vi "Main_v6.vi"() -> ()   [LabVIEW 2018]
uses:
  Clusters/FileDataChannel.ctl
  <vilib>/Platform/TimedLoop/XDataNode/timing_clust.ctl
  <vilib>/Platform/TimedLoop/XDataNode/nitl_modes.ctl
  <vilib>/Platform/TimedLoop/XDataNode/wakeup.ctl
  Clusters/IOSignals.ctl
  Clusters/SimulationConstants.ctl
  Clusters/RoscoParams.ctl
  Clusters/ArrayPairs.ctl
  Clusters/SwapArrayCluster.ctl
  <vilib>/Analysis/baseanly.llb/Mean (DBL).vi
  <vilib>/Utility/file.llb/Read Delimited Spreadsheet (DBL).vi
  <vilib>/Platform/TimedLoop/XDataNode/loadnilvce.vi
  <vilib>/platform/TimedLoop/XDataNode/XDataNode.xnode
  <vilib>/Platform/TimedLoop/XDataNode/XDNodeRunTimeDep.lvlib
  <vilib>/Analysis/NI_AALBase.lvlib
  <vilib>/ptbypt/NI_PtbyPt.lvlib
  <resource>/objmgr/IndComECAT.rc
  <vilib>/indcomecat/Remote IO/NI ECAT Remote IO.lvlib
panel:
  out "State logic late?":bool
  out "Actual shaft Speed (rpm)":dbl(knob)=7.068579725455493e-05 scale=-300.0..300.0
  out "Pitch setpoint (eCAT)":i32
  in  "Man Vel Set":dbl
  in  "Pitch I-Gain":dbl
  in  "Pitch P-Gain":dbl
  out "Main Gen Bus":u16 format="%.0x"
  out "Axis 3 Fault":bool
  out "Axis 3 Warning":bool
  out "Axis 2 Fault":bool
  out "Axis 2 Warning":bool
  out "Axis 1 Fault":bool
  out "Axis 1 Warning":bool
  out "Axis 3 Operational":bool
  out "Axis 2 Operational":bool
  out "Axis 1 Operational":bool
  out "Pitch Axis 3":string
  out "Pitch Axis 2":string
  out "Pitch Axis 1":string
  in  "Clear Pitch Actuator Faults (x3)":bool
  in  "Enable Pitch Actuators (x3)":bool
  out "Pitch Angle (deg) - Blade 3":dbl(knob) scale=0.0..30.0 scale format="%.2f"
  out "Pitch Angle (deg) - Blade 2":dbl(knob) scale=0.0..30.0 scale format="%.2f"
  out "Pitch Angle (deg) - Blade 1":dbl(knob) scale=0.0..30.0 scale format="%.2f"
  in  "Manual Torque":i16(slide) scale=-100.0..250.0
  out "Generator Operational":bool
  in  "Clear Accelnet Faults":bool
  in  "Enable Accelnet":bool
  out "Generator Fault":bool
  out "Generator Warning":bool
  out "Main generator state":string
  out "Rosco Failed?":bool
  in  "WS Freq (Hz)":dbl=0.009999999776482582
  in  "WS Mean":dbl=10.0
  in  "WS Amplitude":dbl
  out "Generator Torque (MNm)":dbl(knob) scale=0.0..35.0
  out "OUT_ROTSP":dbl
  out "OUT_AEROTQ":dbl
  out "SIM-Cp":dbl
  out "Generator Speed (rpm)":dbl(knob)=7.068579725455493e-05 scale=0.0..10.0
  in  "?":T1(tab)
  out "Generator Speed":dynamicdata(graph)
  out "Torque  (MNm)":dynamicdata(graph)
  out "Pitch (deg)":dynamicdata(graph)
  out "Aero Torque":dynamicdata(graph)
  out "WindSpeed(m/s)":dbl(graph)
  in  "To VS_ControlMode":T2(ring)
  in  "Edit DISCON":bool
  out "DISCON.IN Contents":string
  in  "From VS_ControlMode":T2(ring)
  out "Rosco Return Message":string
  out "Generator  Power (kW)":dbl(graph)
  out "Pitch axis 3 ctrl word":u16 format="%x"
  out "Pitch axis 2 ctrl word":u16 format="%x"
  out "avrSWAP":sgl[](array[numeric])
  out "OUT_DEBUG":dbl
  out "RT Loop Duration":i64
  out "Control Mode - Main Gen":u8
  out "WriteSDO Abort - Main Gen":u32
  out "ReadSDO Abort - Main Gen":u32
  out "Gen ctrl word":u16 format="%x"
  out "Pitch axis 1 ctrl word":u16 format="%x"
  out "Graphics Update t (s)":dbl format="%.1f"
  out "Effective rate (ms)":dbl format="%#.1f"
  out "WriteSDO Abort - Pitch 1":u32
  out "ReadSDO Abort - Pitch 1":u32
  out "Control Mode - Pitch 1":u8
  in  "Zero Pitch 1":bool
  in  "Zero Pitch 2":bool
  in  "Zero Pitch 3":bool
  out "Torque Setpoint (MNm)":dbl(knob) scale=0.0..35.0
  out "Collective pitch Setpoint (deg)":dbl(knob) scale=0.0..30.0 scale format="%.2f"
  out "Power (kW)":dbl(slide) scale=0.0..20.0 scale format="%.2f"
  out "SimLoop Late?":bool
  out "FIFO Loop Late?":bool
  in  "Base filename":string="rosco-tests"
  out "Writing to cRIO?":bool
  in  "WriteData":bool
  in  "?":T3
  out "#RT FIFO":u32
  in  "?":bool
  out "Time(s)":dbl format="%6.1g"
  out "RT Loop Late?":bool
  # "FOCAL Campaign 1"
  # "ROSCO"
  # "Processed quantities"
  # "GENERATOR INPUTS"
  # "PITCH ACTUATORS"
  # "FILEWRITING"
  # "MAIN GEN CONTROL"
  # "TEMP"
  # "PITCH ACTUATORS CONTROL"
  # "Axis 1"
  # "Axis 2"
  # "Axis 3"
  # "Operational"
  # "Warning"
  # "Error"
  # "TURBINE SPECIFICATIONS"
  # "RATED POWER: 15000000 W"
  # "RATED TORQUE: 19624046.66 Nm"
  # "RATED GEN SPEED: 0.79168 rad/s"
  # "ROSCO INPUTS"
  # "SYSTEM"
  # "ROSCO"
  # "MAIN MOTOR"
  # "PITCH AXIS 1"
  # "PITCH AXIS 2"
  # "PITCH AXIS 3"
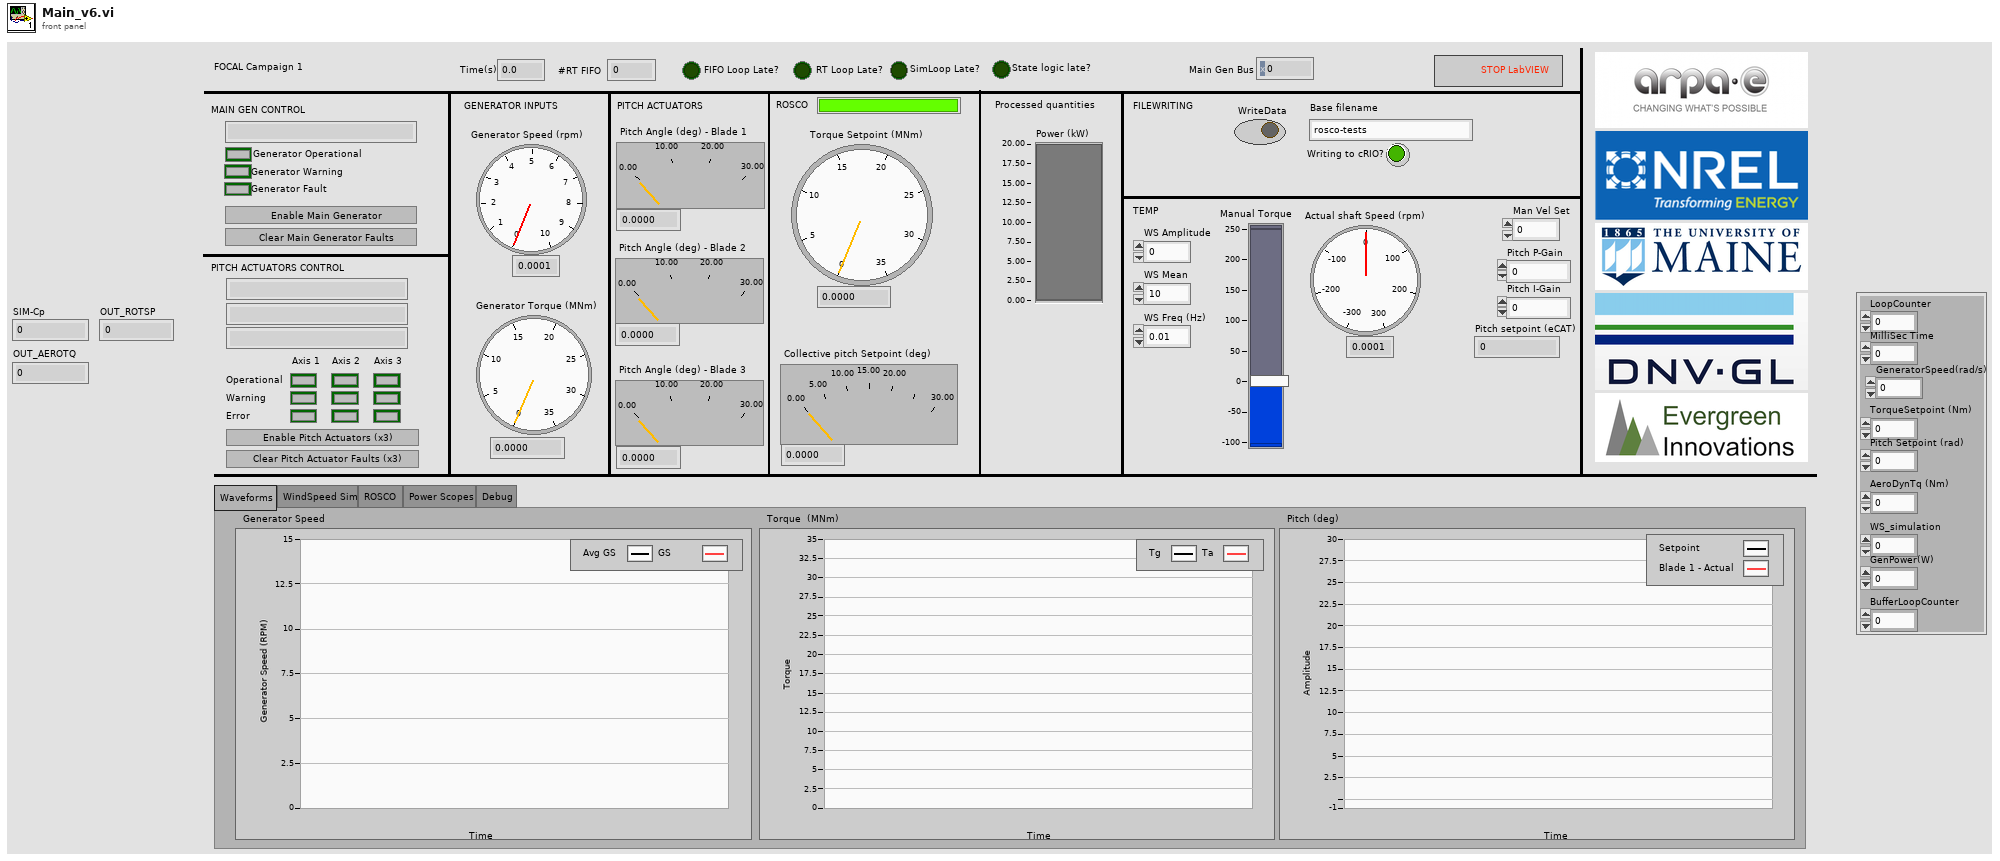
[diagram p1: front panel]
types:
  T1 = enum32{"Waveforms", "WindSpeed Sim", "ROSCO", "Power Scopes", "Debug"}
  T2 = enum16{"Constant Torque", "Constant Power", "PI Control"}
  T3 = typedef "FileDataChannel.ctl" = cluster{"GeneratorSpeed(rad/s)":dbl, "BufferLoopCounter":dbl, "LoopCounter":dbl, "TorqueSetpoint (Nm)":dbl, "Pitch Setpoint (rad)":dbl, "AeroDynTq (Nm) ":dbl, "WS_simulation":dbl, "GenPower(W)":dbl, "MilliSec Time ":dbl}
  T4 = typedef "IOSignals.ctl" = cluster{"mainGenPosition (rev)":dbl, "mainGenTorque (Nm)":dbl, "mainGenVelocity (rpm)":dbl, "mainGenStatus":u16, "pitch1Position (rev)":dbl, "pitch1Velocity (rev/s)":dbl, "pitch1Status":u16, "pitch2Position (rev)":dbl, "pitch2Velocity (rev/s)":dbl, "pitch2Status":u16, "pitch3Position (rev)":dbl, "pitch3Velocity (rev/s)":dbl, "pitch3Status":u16, "pitch1PosOfst (rev)":dbl, "pitch2PosOfst (rev)":dbl, "pitch3PosOfst (rev)":dbl}
  T5 = typedef "ArrayPairs.ctl" = cluster{"iStatus":T6, "TIME":T6, "DT":T6, "BL_PITCH":T6, "VS_MECHGENPWR":T6, "VS_GENPWR":T6, "GEN_SPEED":T6, "ROTOR_SPEED":T6, "GENTQMEAS":T6, "Y_M":T6, "HORWINDV":T6, "ROOTMOOP1":T6, "ROOTMOOP2":T6, "BL_PITCH2":T6, "BL_PITCH3":T6, "ROOTMOOP3":T6, "AVCMSG_SIZE":T6, "INFILE_SIZE ":T6, "OUTFILE_SIZE ":T6, "FA_ACC":T6, "NUM_BLADES":T6, "OUT_BL_PITCH":T6, "OUT_TORQUE":T6, "OUT_AEROTQ":T6, "Out.RotSpeed ":T6, "Out.DEBUG":T6}
  T6 = typedef "SwapArrayCluster.ctl" = cluster{"Index":i32, "Value":dbl}
  T7 = typedef "RoscoParams.ctl" = cluster{"avrSWAP":sgl[], "aviFAIL":i32, "avcMSG":string, "ReturnValue":i32}
  T8 = typedef "XDNodeRunTimeDep.lvlib/timing_clust.ctl" = cluster{"Expected End [f-1]":u64, "Actual End [f-1]":u64, "Finished Late? [f-1]":bool, "Expected End [i-1]":u64, "Actual End [i-1]":u64, "Finished Late? [i-1]":bool, "Expected Start [i]":u64, "Actual Start [i]":u64, "Expected Start [f]":u64, "Actual Start [f]":u64, "Source Name":string, "Structure Name":string, "Period":i64, "Deadline":i64, "Offset":i64, "Start":i64, "Priority":i32, "Timeout":i32, "Mode":T9, "Wakeup Reason":T10, "Error":errorcluster, "Source Type":string, "Secondary Source Type":string, "Global End Time":u64, "Global Start Time":u64, "Frame Duration":u64, "Iteration Duration":u64, "Assigned CPU":i32, "I/O Scan Engine Mode":u32}
  T9 = typedef "XDNodeRunTimeDep.lvlib/nitl_modes.ctl" = enum32{"No Change", "Process missed periods, maintain original phase", "Discard missed periods, maintain original phase", "Process missed periods, ignore original phase", "Discard missed periods, ignore original phase"}
  T10 = typedef "XDNodeRunTimeDep.lvlib/wakeup.ctl" = enum32{"Normal", "Aborted", "Asynchronous wakeup", "Timing source error", "Timed loop error", "Timeout"}
  T11 = typedef "SimulationConstants.ctl" = cluster{"Ngear":dbl, "RotorInertia":dbl, "GeneratorEff":dbl, "RotorRadius":sgl, "Rho":dbl, "NumBlades":dbl, "AVCMSG_SIZE":dbl}
  T12 = typedef "ElmoState.ctl" = cluster{"Elmo State":string, "Elmo Operational":bool, "Elmo Warning":bool, "Elmo Fault":bool}
  T13 = typedef "AccelnetState.ctl" = cluster{"State String":string, "Accelnet Warning":bool, "Accelnet Fault":bool, "Accelnet Operational":bool}
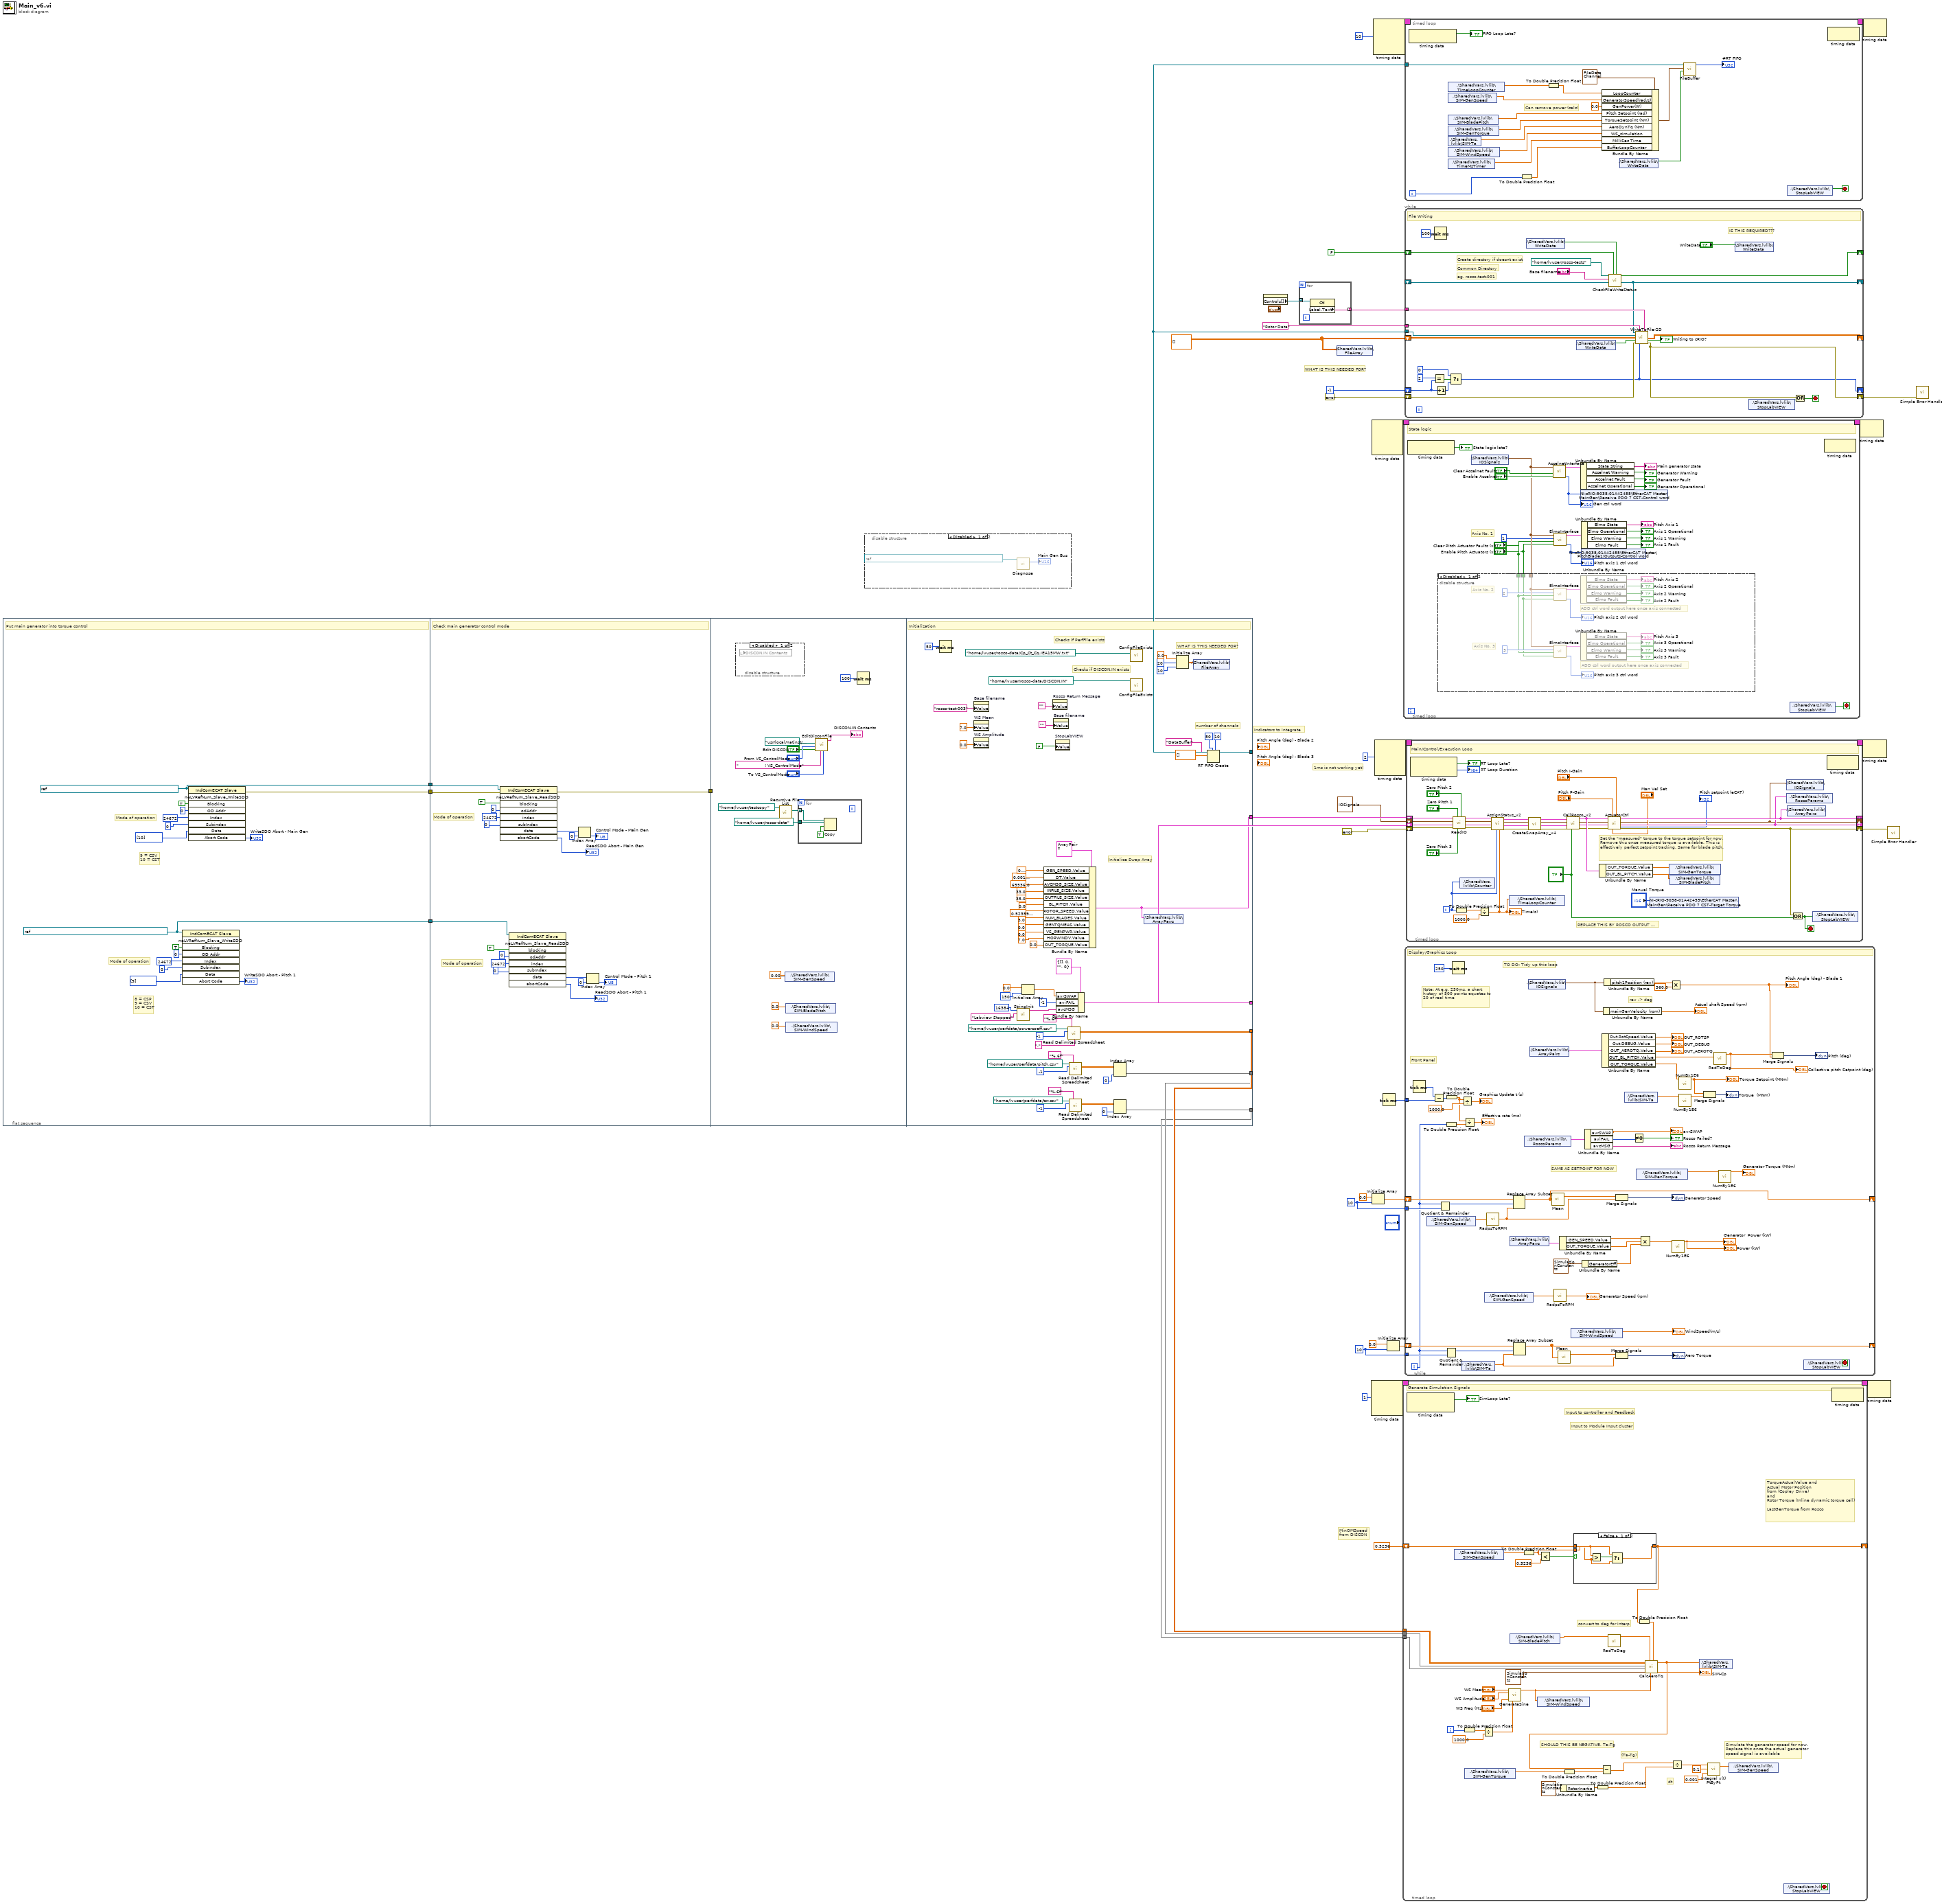
[diagram p0: block diagram]
diagram:
  w16 = 10 ("dimension size")
  w13 = 10 ("dimension size")
  w31 = dbl[][] [] ("File array 2")
  # "Indicators to integrate"
  # "WHAT IS THIS NEEDED FOR?"
  # "1ms is not working yet!"
  # "MinOMSpeed\nfrom DISCON"
  n1 = flat-sequence {
    tunnel: [w48] -> w10
    tunnel: [w49] -> w9
    tunnel: [w41] -> w1
    tunnel: w10 -> [w67]
    tunnel: w9 -> [w66]
    tunnel: [w65] -> w8
    tunnel: w1 -> [w56]
    tunnel: w8 -> [_]
    tunnel: [w140] -> w4
    tunnel: [w129] -> w24
    tunnel: [w105] -> w23
    tunnel: [w118] -> w22
    tunnel: [w117] -> w21
    tunnel: [w92] -> w15
    frame #0 {
      w41 = refnum<k21> "ni.var.io://ni-crio-9038-01a42455/EtherCAT Master/PitchBlade1" ("Slave Constant")
      w48 = refnum<k21> "ni.var.io://ni-crio-9038-01a42455/EtherCAT Master/MainGen" ("Slave Constant")
      # "Mode of operation"
      # "8 = CSP \n9 = CSV\n10 = CST"
      # "Mode of operation"
      # "9 = CSV\n10 = CST"
      # "Put main generator into torque control"
      n2 = invoke class="IndComECAT Slave" method="neLVRefNum_Slave_WriteSDO"(reference=w41, "Blocking"=TRUE, "OD Addr"=u16 0, "Index"=u16 24672, "Subindex"=u8 0, "Data"=u8[] [9]) -> ("Abort Code"=→"WriteSDO Abort - Pitch 1":u32)  [unwired: 3 in, 8 out]
      n3 = invoke class="IndComECAT Slave" method="neLVRefNum_Slave_WriteSDO"(reference=w48, "Blocking"=TRUE, "OD Addr"=u16 0, "Index"=u16 24672, "Subindex"=u8 0, "Data"=u8[] [10]) -> (error out=w49:errorcluster, "Abort Code"=→"WriteSDO Abort - Main Gen":u32)  [unwired: 3 in, 7 out]
    }
    frame #1 {
      # "Mode of operation"
      # "Mode of operation"
      # "Check main generator control mode"
      n4 = invoke class="IndComECAT Slave" method="neLVRefNum_Slave_ReadSDO"(reference=w67, error in=w66, "blocking"=TRUE, "odAddr"=u16 0 ("OD address"), "index"=u16 24672 ("Index"), "subIndex"=u8 0 ("Subindex")) -> (error out=w65:errorcluster, "data"=w70:u8[], "abortCode"=→"ReadSDO Abort - Main Gen":u32)  [unwired: 3 in, 6 out]
      n5 = invoke class="IndComECAT Slave" method="neLVRefNum_Slave_ReadSDO"(reference=w56, "blocking"=TRUE, "odAddr"=u16 0 ("OD address"), "index"=u16 24672 ("Index"), "subIndex"=u8 0 ("Subindex")) -> ("data"=w59:u8[], "abortCode"=→"ReadSDO Abort - Pitch 1":u32)  [unwired: 4 in, 7 out]
      n6 = Index Array(array=w70, index=0) -> (element=→"Control Mode - Main Gen":u8)
      n7 = Index Array(array=w59, index=0) -> (element=→"Control Mode - Pitch 1":u8)
    }
    frame #2 {
      n8 = disable-structure shown="Disabled" {
        frame Disabled {
          n9 = local read "DISCON.IN Contents"() -> ()  [unwired: 1 in]
        }
        frame Enabled {
        }
      }
      n10 = call <vilib>:"Recursive File List.vi"("Folder Path"=path "/home/lvuser/testcopy" ("path")) -> ("All Files in Dir"=w78:path[])  [unwired: 6 in, 4 out]
      n11 = shared-variable ".\\SharedVars.lvlib\\SIM-GenSpeed"(0.009999999776482582 ("RotorSpeed(rad/s)")) -> ()  [unwired: 1 in, 1 out]
      n12 = shared-variable ".\\SharedVars.lvlib\\SIM-BladePitch"(0.0 ("ecat-BladePitch")) -> ()  [unwired: 1 in, 1 out]
      n13 = shared-variable ".\\SharedVars.lvlib\\SIM-WindSpeed"(0.0 ("WindSpeedSim")) -> ()  [unwired: 1 in, 1 out]
      n14 = for {
        tunnel: path "/home/lvuser/rosco-data" ("target path (use dialog)") -> [w91]
        tunnel: w78 -> [w90] mode=indexing
        n15 = Copy(9:TRUE ("overwrite (F)"), 10:w91, 11:w90) -> ()  [unwired: 2 in, 3 out]
      }
      n16 = call "EditDisconFile.vi"("To VS_ControlMode"="To VS_ControlMode", "Append"="                   ! VS_ControlMode", "Edit DISCON"="Edit DISCON", "From VS_ControlMode"="From VS_ControlMode", "path"=path "/usr/local/natinst/labview/DISCON.IN") -> ("data"=→"DISCON.IN Contents":string)  [unwired: 4 in, 1 out]
      n17 = Wait (ms)(milliseconds to wait=u32 100) -> ()  [unwired: 1 out]
    }
    frame #3 {
      # "WHAT IS THIS NEEDED FOR?"
      # "number of channels"
      # "Checks if PerfFile exists"
      # "Checks if DISCON.IN exists"
      # "Initialize Swap Array"
      # "Initialization"
      n18 = Wait (ms)(milliseconds to wait=u32 50) -> ()  [unwired: 1 out]
      n19 = property on="Base filename" class="Str"("Value"="rosco-test-003" ("Base filename")) -> ()  [unwired: 2 in, 2 out]
      n20 = property on="WS Mean" class="DigNum (strict)"("Value"=7.0 ("GenSpeed Mean")) -> ()  [unwired: 2 in, 2 out]
      n21 = property on="WS Amplitude" class="DigNum (strict)"("Value"=0.0 ("GenSpeeed Amplitude")) -> ()  [unwired: 2 in, 2 out]
      n22 = call "StringInit.vi"("accOUTNAME"="Labview Stopped", "dimension size"=16384) -> ("result string"=w144:string)  [unwired: 9 in]
      n23 = Initialize Array(sgl 0.0 ("element"), 150 ("dimension size")) -> (w98:sgl[])
      n24 = Bundle By Name(cluster=T5 {"iStatus"={"Index"=0, "Value"=0.0}, "TIME"={"Index"=1, "Value"=0.0}, "DT"={"Index"=2, "Value"=0.0}, "BL_PITCH"={"Index"=3, "Value"=0.0}, "VS_MECHGENPWR"={"Index"=13, "Value"=0.0}, "VS_GENPWR"={"Index"=14, "Value"=0.0}, "GEN_SPEED"={"Index"=19, "Value"=0.0}, "ROTOR_SPEED"={"Index"=20, "Value"=0.0}, "GENTQMEAS"={"Index"=22, "Value"=0.0}, "Y_M"={"Index"=23, "Value"=0.0}, "HORWINDV"={"Index"=26, "Value"=0.0}, "ROOTMOOP1"={"Index"=29, "Value"=0.0}, "ROOTMOOP2"={"Index"=30, "Value"=0.0}, "BL_PITCH2"={"Index"=32, "Value"=0.0}, "BL_PITCH3"={"Index"=33, "Value"=0.0}, "ROOTMOOP3"={"Index"=31, "Value"=0.0}, "AVCMSG_SIZE"={"Index"=48, "Value"=0.0}, "INFILE_SIZE "={"Index"=49, "Value"=0.0}, "OUTFILE_SIZE "={"Index"=50, "Value"=0.0}, "FA_ACC"={"Index"=52, "Value"=0.0}, "NUM_BLADES"={"Index"=60, "Value"=0.0}, "OUT_BL_PITCH"={"Index"=44, "Value"=0.0}, "OUT_TORQUE"={"Index"=46, "Value"=0.0}, "OUT_AEROTQ"={"Index"=91, "Value"=0.0}, "Out.RotSpeed "={"Index"=92, "Value"=0.0}, "Out.DEBUG"={"Index"=93, "Value"=0.0}} ("ArrayPairs"), "GEN_SPEED.Value"=0.30000001192092896 ("GeneratorSpeed(rad/s)"), "DT.Value"=0.0010000000474974513 ("Dt"), "AVCMSG_SIZE.Value"=65536.0 ("new element/subarray"), "INFILE_SIZE.Value"=33.0 ("new element/subarray"), "OUTFILE_SIZE.Value"=35.0 ("new element/subarray"), "BL_PITCH.Value"=0.0 ("GeneratorTorque(Nm)"), "ROTOR_SPEED.Value"=0.5235999822616577 ("RotorSpeed(rad/s)"), "NUM_BLADES.Value"=3.0 ("NumberofBlades"), "GENTQMEAS.Value"=0.0 ("BladePitch(rad)"), "VS_GENPWR.Value"=0.0 ("Generator Power(W)"), "HORWINDV.Value"=7.0 ("WindSpeed(m/s)"), "OUT_TORQUE.Value"=0.0) -> (w92:T5)
      n25 = property on="Rosco Return Message" class="Str"("Value"="") -> ()  [unwired: 2 in, 2 out]
      n26 = property on="Base filename" class="Str"("Value"="") -> ()  [unwired: 2 in, 2 out]
      n27 = property on="StopLabVIEW" class="Bool (strict)"("Value"=FALSE) -> ()  [unwired: 2 in, 2 out]
      n28 = Bundle By Name(cluster=T7 {"avrSWAP"=[], "aviFAIL"=0, "avcMSG"="", "ReturnValue"=0}, "avrSWAP"=w98, "aviFAIL"=-1, "avcMSG"=w144) -> (w129:T7)
      n29 = call-poly <vilib>:"Read Delimited Spreadsheet.vi"("file path (dialog if empty)"=path "/home/lvuser/perfdata/powercoeff.csv", "format (%.3f)"="%.6f", "number of rows (all:-1)"=-1, "delimiter (\\t)"="," ("delimiter (\\t)")) -> ("all rows"=w105:dbl[][])  [unwired: 6 in, 5 out]
      n30 = call-poly <vilib>:"Read Delimited Spreadsheet.vi"("file path (dialog if empty)"=path "/home/lvuser/perfdata/pitch.csv", "format (%.3f)"="%.6f", "number of rows (all:-1)"=-1) -> ("all rows"=w122:dbl[][])  [unwired: 7 in, 5 out]
      n31 = call-poly <vilib>:"Read Delimited Spreadsheet.vi"("file path (dialog if empty)"=path "/home/lvuser/perfdata/tsr.csv", "format (%.3f)"="%.6f", "number of rows (all:-1)"=-1) -> ("all rows"=w124:dbl[][])  [unwired: 7 in, 5 out]
      n32 = Index Array(array=w122, index (col)=0 ("disabled index (col)")) -> (element=w118:dbl[])  [unwired: 1 in]
      n33 = Index Array(array=w124, index (col)=0 ("disabled index (col)")) -> (element=w117:dbl[])  [unwired: 1 in]
      n34 = call "ConfigFileExists.vi"("path"=path "/home/lvuser/rosco-data/Cp_Ct_Cq.IEA15MW.txt") -> ()  [unwired: 11 in]
      n35 = call "ConfigFileExists.vi"("path"=path "/home/lvuser/rosco-data/DISCON.IN") -> ()  [unwired: 11 in]
      n36 = shared-variable ".\\SharedVars.lvlib\\ArrayPairs"(w92) -> ()  [unwired: 1 in, 1 out]
      n37 = Initialize Array(0.0 ("element"), 20 ("dimension size"), 10 ("dimension size")) -> (w136:dbl[][])
      n38 = shared-variable ".\\SharedVars.lvlib\\FileArray"(w136) -> ()  [unwired: 1 in, 1 out]
      n39 = RT FIFO Create(0:"DataBuffer" ("name (unnamed)"), 1:dbl[] [] ("appended array"), 4:u32 50, 6:u32 10) -> (8:w140:refnum<k33>)  [unwired: 4 in, 2 out]
    }
  }
  n40 = disable-structure shown="Disabled" {
    frame Disabled {
      n41 = call <vilib>:"Diagnose.vi"("slave reference in"=refnum<k21> "ni.var.io://ni-crio-9038-01a42455/EtherCAT Master/MainGen" ("Slave Constant")) -> ("bus state"=→"Main Gen Bus":u16)  [unwired: 10 in, 4 out]
    }
    frame Enabled {
    }
  }
  n42 = property class="Clust (strict)"() -> ("Controls[]"=w34:refnum<vi>[])  [unwired: 2 in, 2 out]
  n43 = for {
    tunnel: w34 -> [w153] mode=indexing
    tunnel: [w152] -> w33 mode=indexing
    n44 = property class="Ctl"(reference=w153) -> ("Label.Text"=w152:string)  [unwired: 1 in, 2 out]
  }
  n45 = shared-variable ".\\SharedVars.lvlib\\FileArray"(w31) -> ()  [unwired: 1 in, 1 out]
  n46 = node-c288(i64 1 ("Period")) -> (w40:T8)  [unwired: 3 in]
  n47 = node-c288() -> (w12:T8)  [unwired: 4 in]
  n48 = Initialize Array(0.0 ("element"), w13) -> (w19:dbl[])
  n49 = node-c288(i64 10 ("Period")) -> (w7:T8)  [unwired: 3 in]
  n50 = node-c288(i64 2 ("Period")) -> (w38:T8)  [unwired: 3 in]
  n51 = Tick Count (ms)() -> (millisecond timer value=w2:u32)
  n52 = Initialize Array(0.0 ("element"), w16) -> (w17:dbl[])
  n53 = timed-loop {
    timing: w40 -> [_]
    timing-out: [_] -> w39
    tunnel: w23 -> [w186]
    tunnel: w22 -> [w185]
    tunnel: w21 -> [w184]
    shift-right: [w156] -> _
    shift-left: 0.5236 -> [w158]
    i -> [w167]
    stop <- w188 stop-if-true
    # "Simulate the generator speed for now. Replace this once the actual generator speed signal is available"
    # "dt"
    # "SHOULD THIS BE NEGATIVE, Ta-Tg"
    # "(Ta-Tg)"
    # "convert to deg for interp"
    # "TorqueActualValue and \nActual Motor Position \nfrom (Copley Drive)\nand\nRotor Torque (Inline dynamic torque cell)\n\nLastGenTorque from Rosco"
    # "Input to Module Input cluster"
    # "Input to controller and Feedback"
    # "Generate Simulation Signals"
    n54 = node-c288() -> (→"SimLoop Late?":bool)  [unwired: 1 in, 1 out]
    n55 = shared-variable ".\\SharedVars.lvlib\\SIM-GenSpeed"() -> (w161:dbl)  [unwired: 1 in, 1 out]
    n56 = To Double Precision Float(number=w167) -> (double precision float=w166:dbl)
    n57 = shared-variable ".\\SharedVars.lvlib\\SIM-GenTorque"() -> (w172:dbl)  [unwired: 1 in, 1 out]
    n58 = Divide(x=w166, y=1000.0) -> (x/y=w177:dbl)
    n59 = call "GenerateSine.vi"("GenSpeed Mean"="WS Mean", "GenSpeeed Amplitude"="WS Amplitude", "frequency (f)"="WS Freq (Hz)", "time (s)"=w177) -> ("sine out"=w165:dbl)  [unwired: 11 in]
    n60 = shared-variable ".\\SharedVars.lvlib\\SIM-BladePitch"() -> (w154:dbl)  [unwired: 1 in, 1 out]
    n61 = To Double Precision Float(number=w161) -> (double precision float=w157:dbl)
    n62 = shared-variable ".\\SharedVars.lvlib\\SIM-WindSpeed"(w165) -> ()  [unwired: 1 in, 1 out]
    n63 = Less?(x=w157, y=0.5236) -> (x < y?=w159:bool)
    n64 = Unbundle By Name(T11 {"Ngear"=1.0, "RotorInertia"=318628128.0, "GeneratorEff"=0.9700000286102295, "RotorRadius"=120.0, "Rho"=1.225000023841858, "NumBlades"=1.225000023841858, "AVCMSG_SIZE"=1.225000023841858} ("SimulationConst")) -> ("RotorInertia"=w175:dbl)
    n65 = To Double Precision Float(number=w172) -> (double precision float=w173:dbl)
    n66 = case shown="False" w159 {
      tunnel: [w189 w193] -> w156
      tunnel: w158 -> [w190 w193]
      tunnel: w157 -> [w191 _]
      frame False {
        n67 = Greater?(x=w191, y=w190) -> (0:w192:bool)
        n68 = Select(t=w191, s=w192, f=w190) -> (s? t:f=w189:dbl)
      }
      frame True {
      }
    }
    n69 = To Double Precision Float(number=w175) -> (double precision float=w171:dbl)
    n70 = call "RadToDeg.vi"("Double"=w154) -> ("Numeric"=w164:dbl)  [unwired: 10 in]
    n71 = To Double Precision Float(number=w156) -> (double precision float=w176:dbl)
    n72 = call "CalcAeroTq.vi"("GenSpeed"=w176, "WindSpeed"=w165, "Xi"=w164, "SimulationConst"=T11 {"Ngear"=1.0, "RotorInertia"=318628128.0, "GeneratorEff"=0.9700000286102295, "RotorRadius"=120.0, "Rho"=1.225000023841858, "NumBlades"=1.225000023841858, "AVCMSG_SIZE"=1.225000023841858}, "tsr(Y)"=w184, "pitch (X)"=w185, "Cp(Z)"=w186) -> ("Cp"=→"SIM-Cp":dbl, "Ta"=w163:dbl)  [unwired: 2 in]
    n73 = Subtract(x=w163, y=w173) -> (x-y=w162:dbl)
    n74 = Divide(x=w162, y=w171) -> (x/y=w170:dbl)
    n75 = shared-variable ".\\SharedVars.lvlib\\SIM-Ta"(w163) -> ()  [unwired: 1 in, 1 out]
    n76 = call <vilib>:"Integral x(t) PtByPt.vi"("dt"=0.001, "initial condition"=0.1, "x"=w170) -> ("integral x(t)"=w155:dbl)  [unwired: 1 in, 1 out]
    n77 = shared-variable ".\\SharedVars.lvlib\\SIM-GenSpeed"(w155) -> ()  [unwired: 1 in, 1 out]
    n78 = shared-variable ".\\SharedVars.lvlib\\StopLabVIEW"() -> (w188:bool)  [unwired: 1 in, 1 out]
    n79 = node-c288() -> ()  [unwired: 1 in, 1 out]
  }
  n80 = timed-loop {
    timing: w12 -> [_]
    timing-out: [_] -> w11
    stop <- w216 stop-if-true
    # "Axis No. 1"
    # "State logic"
    n81 = node-c288() -> (→"State logic late?":bool)  [unwired: 1 in]
    n82 = shared-variable ".\\SharedVars.lvlib\\IOSignals"() -> (w207:T4)  [unwired: 1 in, 1 out]
    n83 = disable-structure shown="Disabled" {
      disable-tunnel: w207 -> [w233 _]
      disable-tunnel: "Clear Pitch Actuator Faults (x3)" -> [w229 _]
      disable-tunnel: "Enable Pitch Actuators (x3)" -> [w228 _]
      frame Disabled {
        # "ADD ctrl word output here once axis connected"
        # "ADD ctrl word output here once axis connected"
        # "Axis No. 3"
        # "Axis No. 2"
        n84 = call "ElmoInterface.vi"("Enable"=w228, "Clear faults"=w229, "Axis No."=u32 2, "IO Signals"=w233) -> ("Control word"=→"Pitch axis 2 ctrl word":u16, "Elmo State Cluster Out"=w231:T12)  [unwired: 6 in]
        n85 = call "ElmoInterface.vi"("Enable"=w228, "Clear faults"=w229, "Axis No."=u32 3, "IO Signals"=w233) -> ("Control word"=→"Pitch axis 3 ctrl word":u16, "Elmo State Cluster Out"=w227:T12)  [unwired: 6 in]
        n86 = Unbundle By Name(w231) -> ("Elmo State"=→"Pitch Axis 2":string, "Elmo Operational"=→"Axis 2 Operational":bool, "Elmo Warning"=→"Axis 2 Warning":bool, "Elmo Fault"=→"Axis 2 Fault":bool)
        n87 = Unbundle By Name(w227) -> ("Elmo State"=→"Pitch Axis 3":string, "Elmo Operational"=→"Axis 3 Operational":bool, "Elmo Warning"=→"Axis 3 Warning":bool, "Elmo Fault"=→"Axis 3 Fault":bool)
      }
      frame Enabled {
      }
    }
    n88 = call "AccelnetInterface.vi"("Enable"="Enable Accelnet", "Clear Faults"="Clear Accelnet Faults", "IO Signals"=w207) -> ("Control word"=w211:u16, "Accelnet State"=w215:T13)  [unwired: 7 in]
    "Gen ctrl word" <- w211
    n89 = call "ElmoInterface.vi"("Enable"="Enable Pitch Actuators (x3)", "Clear faults"="Clear Pitch Actuator Faults (x3)", "Axis No."=u32 1, "IO Signals"=w207) -> ("Control word"=w198:u16, "Elmo State Cluster Out"=w206:T12)  [unwired: 6 in]
    "Pitch axis 1 ctrl word" <- w198
    n90 = Unbundle By Name(w215) -> ("State String"=→"Main generator state":string, "Accelnet Warning"=→"Generator Warning":bool, "Accelnet Fault"=→"Generator Fault":bool, "Accelnet Operational"=→"Generator Operational":bool)
    n91 = shared-variable "NI-cRIO-9038-01A42455\\EtherCAT Master\\MainGen\\Receive PDO 7 CST-Control word"(w211) -> ()  [unwired: 1 in, 1 out]
    n92 = Unbundle By Name(w206) -> ("Elmo State"=→"Pitch Axis 1":string, "Elmo Operational"=→"Axis 1 Operational":bool, "Elmo Warning"=→"Axis 1 Warning":bool, "Elmo Fault"=→"Axis 1 Fault":bool)
    n93 = shared-variable "NI-cRIO-9038-01A42455\\EtherCAT Master\\PitchBlade1\\Outputs-Control word"(w198) -> ()  [unwired: 1 in, 1 out]
    n94 = shared-variable ".\\SharedVars.lvlib\\StopLabVIEW"() -> (w216:bool)  [unwired: 1 in, 1 out]
    n95 = node-c288() -> ()  [unwired: 1 in, 1 out]
  }
  n96 = timed-loop {
    timing: w7 -> [_]
    timing-out: [_] -> w6
    tunnel: w4 -> [w238]
    i -> [w237]
    stop <- w239 stop-if-true
    # "Can remove power (calc)"
    n97 = node-c288() -> (→"FIFO Loop Late?":bool)  [unwired: 1 in]
    n98 = shared-variable ".\\SharedVars.lvlib\\TimeLoopCounter"() -> (w245:dbl)  [unwired: 1 in, 1 out]
    n99 = shared-variable ".\\SharedVars.lvlib\\SIM-GenSpeed"() -> (w253:dbl)  [unwired: 1 in, 1 out]
    n100 = shared-variable ".\\SharedVars.lvlib\\SIM-BladePitch"() -> (w247:dbl)  [unwired: 1 in, 1 out]
    n101 = shared-variable ".\\SharedVars.lvlib\\SIM-GenTorque"() -> (w248:dbl)  [unwired: 1 in, 1 out]
    n102 = shared-variable ".\\SharedVars.lvlib\\SIM-Ta"() -> (w249:dbl)  [unwired: 1 in, 1 out]
    n103 = shared-variable ".\\SharedVars.lvlib\\SIM-WindSpeed"() -> (w250:dbl)  [unwired: 1 in, 1 out]
    n104 = shared-variable ".\\SharedVars.lvlib\\TimeMsTimer"() -> (w251:dbl)  [unwired: 1 in, 1 out]
    n105 = To Double Precision Float(number=w237) -> (double precision float=w246:dbl)
    n106 = To Double Precision Float(number=w245) -> (double precision float=w240:dbl)
    n107 = Bundle By Name(cluster=T3 {"GeneratorSpeed(rad/s)"=0.0, "BufferLoopCounter"=0.0, "LoopCounter"=0.0, "TorqueSetpoint (Nm)"=0.0, "Pitch Setpoint (rad)"=0.0, "AeroDynTq (Nm) "=0.0, "WS_simulation"=0.0, "GenPower(W)"=0.0, "MilliSec Time "=0.0} ("SwapIn"), "LoopCounter"=w240, "GeneratorSpeed(rad/s)"=w253, "GenPower(W)"=0.0, "Pitch Setpoint (rad)"=w247, "TorqueSetpoint (Nm)"=w248, "AeroDynTq (Nm)"=w249, "WS_simulation"=w250, "MilliSec Time"=w251, "BufferLoopCounter"=w246) -> (w242:T3)
    n108 = shared-variable ".\\SharedVars.lvlib\\WriteData"() -> (w243:bool)  [unwired: 1 in, 1 out]
    n109 = call "FileBuffer.vi"("Boolean"=w243, "FileDataChannel"=w242, "Refnum in"=w238) -> ("# elements"=→"#RT FIFO":u32)  [unwired: 8 in]
    n110 = shared-variable ".\\SharedVars.lvlib\\StopLabVIEW"() -> (w239:bool)  [unwired: 1 in, 1 out]
    n111 = node-c288() -> ()  [unwired: 1 in, 1 out]
  }
  n112 = while {
    shift-right: [w260] -> _
    shift-left: _ -> [w261]
    shift-right: [w268] -> _
    shift-left: FALSE -> [w269]
    shift-right: [w280] -> w27
    shift-left: errorcluster {"status"=FALSE, "code"=0, "source"=""} ("error out") -> [w279]
    tunnel: "Rotor Data" -> [w263]
    tunnel: w33 -> [w264]
    tunnel: w4 -> [w265]
    shift-right: [w276] -> _
    shift-left: -1 -> [w278]
    shift-right: [w271] -> _
    shift-left: w31 -> [w277]
    stop <- w282 stop-if-true
    # "IS THIS REQUIRED???"
    # "eg. rosco-test-001"
    # "Create directory if doesnt exist"
    # "Common Directory"
    # "File Writing"
    n113 = Equal?(x=2 ("t"), y=w278) -> (x = y?=w273:bool)
    n114 = Wait (ms)(milliseconds to wait=u32 100) -> ()  [unwired: 1 out]
    n115 = Increment(x=w278) -> (x+1=w272:i32)
    n116 = Select(t=0, s=w273, f=w272) -> (s? t:f=w276:i32)
    n117 = shared-variable ".\\SharedVars.lvlib\\WriteData"() -> (w270:bool)  [unwired: 1 in, 1 out]
    n118 = shared-variable ".\\SharedVars.lvlib\\WriteData"() -> (w266:bool)  [unwired: 1 in, 1 out]
    n119 = call "CheckFIleWriteStatus.vi"("WriteDataButtonVal"=w270, "WritePrevVal"=w269, "Refnum in"=w261, "Base filename"="Base filename", "File path"=path "/home/lvuser/rosco-tests") -> ("Refnum out"=w260:refnum<k34>, "WriteCurrentVal"=w268:bool)  [unwired: 5 in]
    n120 = call "WriteToFile-2D.vi"("Refnum in"=w260, "Group Name"=w263, "Channel Names"=w264, "rt fifo"=w265, "File array"=w277, "Write?"=w266, "error in (no error)"=w279, "index"=w276) -> ("File array 2"=w271:dbl[][], "Writing to file"=→"Writing to cRIO?":bool, "error out"=w280:errorcluster)  [unwired: 4 in, 1 out]
    n121 = shared-variable ".\\SharedVars.lvlib\\WriteData"("WriteData") -> ()  [unwired: 1 in, 1 out]
    n122 = shared-variable ".\\SharedVars.lvlib\\StopLabVIEW"() -> (w283:bool)  [unwired: 1 in, 1 out]
    n123 = Or(x=w280, y=w283) -> (x .or. y?=w282:bool)
  }
  n124 = while {
    shift-right: [w334] -> _
    shift-left: w19 -> [w336]
    tunnel: w13 -> [w304]
    shift-right: [w331] -> _
    shift-left: w17 -> [w332]
    tunnel: w16 -> [w303]
    tunnel: w2 -> [w294]
    i -> [w288]
    stop <- w343 stop-if-true
    # "rev -> deg"
    # "TO DO: Tidy up this loop"
    # "SAME AS SETPOINT FOR NOW"
    # "Note: At e.g. 250ms, a chart history of 500 points equates to 20 of real time"
    # "Front Panel"
    # "Display/Graphics Loop"
    n125 = Tick Count (ms)() -> (millisecond timer value=w295:u32)
    n126 = shared-variable ".\\SharedVars.lvlib\\SIM-GenSpeed"() -> (w306:dbl)  [unwired: 1 in, 1 out]
    n127 = Subtract(x=w295, y=w294) -> (x-y=w291:u32)
    n128 = Quotient & Remainder(x=w288, y=w304) -> (x-y*floor(x/y)=w335:i32)  [unwired: 1 out]
    n129 = To Double Precision Float(number=w288) -> (double precision float=w289:dbl)
    n130 = Quotient & Remainder(x=w288, y=w303) -> (x-y*floor(x/y)=w333:i32)  [unwired: 1 out]
    n131 = To Double Precision Float(number=w291) -> (double precision float=w290:dbl)
    n132 = Wait (ms)(milliseconds to wait=u32 250 ("Period")) -> ()  [unwired: 1 out]
    n133 = Divide(x=w290, y=1000.0) -> (x/y=→"Graphics Update t (s)":dbl)
    n134 = shared-variable ".\\SharedVars.lvlib\\SIM-Ta"() -> (w327:dbl)  [unwired: 1 in, 1 out]
    n135 = Divide(x=w290, y=w289) -> (x/y=→"Effective rate (ms)":dbl)
    n136 = shared-variable ".\\SharedVars.lvlib\\SIM-GenSpeed"() -> (w308:dbl)  [unwired: 1 in, 1 out]
    n137 = call "RadpsToRPM.vi"("radps"=w306) -> ("rpm"=w305:dbl)
    n138 = shared-variable ".\\SharedVars.lvlib\\ArrayPairs"() -> (w312:T5)  [unwired: 1 in, 1 out]
    n139 = Replace Array Subset(array=w336, new element=w305, index=w335) -> (w334:dbl[])
    n140 = Replace Array Subset(array=w332, new element=w327, index=w333) -> (w331:dbl[])
    n141 = shared-variable ".\\SharedVars.lvlib\\RoscoParams"() -> (w342:T7)  [unwired: 1 in, 1 out]
    n142 = shared-variable ".\\SharedVars.lvlib\\IOSignals"() -> (w286:T4)  [unwired: 1 in, 1 out]
    n143 = shared-variable ".\\SharedVars.lvlib\\ArrayPairs"() -> (w317:T5)  [unwired: 1 in, 1 out]
    n144 = call-poly <vilib>:"Mean.vi"("X"=w334) -> ("mean"=w330:dbl)  [unwired: 1 out]
    n145 = call "RadpsToRPM.vi"("radps"=w308) -> ("rpm"=→"Generator Speed (rpm)":dbl)
    n146 = call-poly <vilib>:"Mean.vi"("X"=w331) -> ("mean"=w328:dbl)  [unwired: 1 out]
    n147 = Unbundle By Name(w312) -> ("GEN_SPEED.Value"=w311:dbl, "OUT_TORQUE.Value"=w310:dbl)
    n148 = shared-variable ".\\SharedVars.lvlib\\SIM-WindSpeed"() -> (→"WindSpeed(m/s)":dbl)  [unwired: 1 in, 1 out]
    n149 = Unbundle By Name(T11 {"Ngear"=1.0, "RotorInertia"=318628128.0, "GeneratorEff"=0.9700000286102295, "RotorRadius"=120.0, "Rho"=1.225000023841858, "NumBlades"=1.225000023841858, "AVCMSG_SIZE"=1.225000023841858} ("SimulationConst")) -> ("GeneratorEff"=w313:dbl)
    n150 = Unbundle By Name(w342) -> ("avrSWAP"=→"avrSWAP":sgl[], "aviFAIL"=w340:i32, "avcMSG"=→"Rosco Return Message":string)
    n151 = Unbundle By Name(w317) -> ("Out.RotSpeed.Value"=→"OUT_ROTSP":dbl, "Out.DEBUG.Value"=→"OUT_DEBUG":dbl, "OUT_AEROTQ.Value"=→"OUT_AEROTQ":dbl, "OUT_BL_PITCH.Value"=w316:dbl, "OUT_TORQUE.Value"=w315:dbl)
    n152 = Unbundle By Name(w286) -> ("mainGenVelocity (rpm)"=→"Actual shaft Speed (rpm)":dbl)
    n153 = Unbundle By Name(w286) -> ("pitch1Position (rev)"=w298:dbl)
    n154 = Merge Signals(w330, w305) -> (→"Generator Speed":dynamicdata)
    n155 = Merge Signals(w328, w327) -> (→"Aero Torque":dynamicdata)
    n156 = shared-variable ".\\SharedVars.lvlib\\SIM-Ta"() -> (w323:dbl)  [unwired: 1 in, 1 out]
    n157 = Not Equal To 0?(x=w340) -> (x != 0?=→"Rosco Failed?":bool)
    n158 = shared-variable ".\\SharedVars.lvlib\\SIM-GenTorque"() -> (w300:dbl)  [unwired: 1 in, 1 out]
    n159 = Compound Arithmetic op=MULTIPLY(w311, w310, w313) -> (w309:dbl)
    n160 = Multiply(x=w298, y=360.0) -> (x*y=w284:dbl)
    "Pitch Angle (deg) - Blade 1" <- w284
    n161 = call "NumBy1E6.vi"("Double"=w309) -> ("Numeric"=→"Power (kW)" →"Generator  Power (kW)":dbl)  [unwired: 10 in]
    n162 = call "NumBy1E6.vi"("Double"=w315) -> ("Numeric"=w324:dbl)  [unwired: 10 in]
    "Torque Setpoint (MNm)" <- w324
    n163 = call "NumBy1E6.vi"("Double"=w323) -> ("Numeric"=w322:dbl)  [unwired: 10 in]
    n164 = Merge Signals(w324, w322) -> (→"Torque  (MNm)":dynamicdata)
    n165 = call "RadToDeg.vi"("Double"=w316) -> ("Numeric"=w301:dbl)  [unwired: 10 in]
    "Collective pitch Setpoint (deg)" <- w301
    n166 = call "NumBy1E6.vi"("Double"=w300) -> ("Numeric"=→"Generator Torque (MNm)":dbl)  [unwired: 10 in]
    n167 = Merge Signals(w301, w284) -> (→"Pitch (deg)":dynamicdata)
    n168 = shared-variable ".\\SharedVars.lvlib\\StopLabVIEW"() -> (w343:bool)  [unwired: 1 in, 1 out]
  }
  n169 = timed-loop {
    timing: w38 -> [_]
    timing-out: [_] -> w37
    shift-right: [w354] -> _
    shift-left: w24 -> [w366]
    shift-right: [w353] -> w25
    shift-left: errorcluster {"status"=FALSE, "code"=0, "source"=""} ("error out") -> [w365]
    shift-right: [w357] -> _
    shift-left: w15 -> [w369]
    shift-right: [w347] -> _
    shift-left: T4 {"mainGenPosition (rev)"=0.0, "mainGenTorque (Nm)"=0.0, "mainGenVelocity (rpm)"=0.0, "mainGenStatus"=0, "pitch1Position (rev)"=0.0, "pitch1Velocity (rev/s)"=0.0, "pitch1Status"=0, "pitch2Position (rev)"=0.0, "pitch2Velocity (rev/s)"=0.0, "pitch2Status"=0, "pitch3Position (rev)"=0.0, "pitch3Velocity (rev/s)"=0.0, "pitch3Status"=0, "pitch1PosOfst (rev)"=0.0, "pitch2PosOfst (rev)"=0.0, "pitch3PosOfst (rev)"=0.0} -> [w363]
    i -> [w370]
    stop <- w382 stop-if-true
    # "REPLACE THIS BY ROSCO OUTPUT ..."
    # "Set the \"measured\" torque to the torque setpoint for now. Remove this once measured torque is available. This is effectively perfect setpoint tracking. Same for blade pitch."
    # "Main/Control/Execution Loop"
    n170 = node-c288() -> (→"RT Loop Late?":bool, →"RT Loop Duration":i64)  [unwired: 1 in]
    n171 = call "ReadIO.vi"("Zero Pitch 2"="Zero Pitch 2", "Zero Pitch 3"="Zero Pitch 3", "Zero Pitch 1"="Zero Pitch 1", "error in"=w365, "ROSCO Params In"=w366, "IO Signals In"=w363, "ArrayPairs In"=w369) -> ("error out"=w364:errorcluster, "ROSCO Params Out"=w367:T7, "IO Signals Out"=w362:T4, "ArrayPairs Out"=w368:T5)  [unwired: 1 in]
    n172 = To Double Precision Float(number=w370) -> (double precision float=w384:dbl)
    n173 = shared-variable ".\\SharedVars.lvlib\\Counter"(w370) -> ()  [unwired: 1 in, 1 out]
    n174 = Divide(x=w384, y=1000.0) -> (x/y=w371:dbl)
    "Time(s)" <- w371
    n175 = call "AssignStatus_v2.vi"("Time (s)"=w371, "LoopCount"=w370, "error in (no error)"=w364, "ROSCO Params In"=w367, "IO Signals In"=w362, "ArrayPairs In"=w368) -> ("error out"=w379:errorcluster, "ROSCO Params Out"=w380:T7, "IO Signals Out"=w360:T4, "ArrayPairs Out"=w381:T5)  [unwired: 2 in]
    n176 = shared-variable ".\\SharedVars.lvlib\\TimeLoopCounter"(w371) -> ()  [unwired: 1 in, 1 out]
    n177 = call "CreateSwapArray_v4.vi"("error in (no error)"=w379, "ROSCO Params"=w380, "IO Signals In"=w360, "ArrayPairs"=w381) -> ("error out"=w376:errorcluster, "ROSCO Params Out"=w377:T7, "IO Signals Out"=w359:T4, "ArrayPairs Out"=w378:T5)  [unwired: 4 in]
    n178 = call "CallRosco_v2.vi"("StopLV"="?", "error in (no error)"=w376, "ROSCO Params in"=w377, "IO Signals In"=w359, "ArrayPairs"=w378) -> ("error out"=w352:errorcluster, "ROSCO Params Out"=w355:T7, "IO Signals Out"=w356:T4, "ArrayPairs Out"=w358:T5)  [unwired: 3 in]
    n179 = Unbundle By Name(w358) -> ("OUT_TORQUE.Value"=w373:dbl, "OUT_BL_PITCH.Value"=w372:dbl)
    n180 = call "ActuatorCtrl.vi"("integral"="Pitch I-Gain", "Man Vel Set (rev/s)"="Man Vel Set", "proportional"="Pitch P-Gain", "error in (no error)"=w352, "ROSCO Params in"=w355, "IO Signals In"=w356, "ArrayPairs In"=w358) -> ("error out"=w353:errorcluster, "ROSCO Params Out"=w354:T7, "IO Signals Out"=w347:T4, "ArrayPairs Out"=w357:T5, "Pitch setpoint (eCAT)"=→"Pitch setpoint (eCAT)":i32)
    n181 = shared-variable "NI-cRIO-9038-01A42455\\EtherCAT Master\\MainGen\\Receive PDO 7 CST-Target Torque"("Manual Torque") -> ()  [unwired: 1 in, 1 out]
    n182 = shared-variable ".\\SharedVars.lvlib\\SIM-GenTorque"(w373) -> ()  [unwired: 1 in, 1 out]
    n183 = shared-variable ".\\SharedVars.lvlib\\SIM-BladePitch"(w372) -> ()  [unwired: 1 in, 1 out]
    n184 = shared-variable ".\\SharedVars.lvlib\\IOSignals"(w347) -> ()  [unwired: 1 in, 1 out]
    n185 = shared-variable ".\\SharedVars.lvlib\\RoscoParams"(w354) -> ()  [unwired: 1 in, 1 out]
    n186 = shared-variable ".\\SharedVars.lvlib\\ArrayPairs"(w357) -> ()  [unwired: 1 in, 1 out]
    n187 = Or(x=w353, y="?") -> (x .or. y?=w382:bool)
    n188 = shared-variable ".\\SharedVars.lvlib\\StopLabVIEW"(w382) -> ()  [unwired: 1 in, 1 out]
    n189 = node-c288() -> ()  [unwired: 1 in, 1 out]
  }
  n190 = node-c288(w11) -> ()  [unwired: 1 out]
  n191 = node-c288(w37) -> ()  [unwired: 1 out]
  n192 = node-c288(w6) -> ()  [unwired: 1 out]
  n193 = node-c288(w39) -> ()  [unwired: 1 out]
  n194 = call <vilib>:"Simple Error Handler.vi"("error in (no error)"=w25) -> ()  [unwired: 4 in, 5 out]
  n195 = call <vilib>:"Simple Error Handler.vi"("error in (no error)"=w27) -> ()  [unwired: 4 in, 5 out]
